vi "rename channel test.vi"() -> ()   [LabVIEW 2013, in "current tag file io module tests.lvlib"]
uses:
  current tag file io module tests.lvlib
  module/configuration/tag configuration.ctl
  <vilib>/NI/Tag Bus Module Framework/channel/TBM channel.lvclass
  <vilib>/NI/Tag Bus/tag/Data Type.ctl
  module/configuration/current tag file io module configuration.lvclass/current tag file io module configuration.ctl
  <vilib>/NI/Tag Bus/tag/tag descriptor.lvclass/tag descriptor.ctl
  module/configuration/Read tags.vi
  module/configuration/current tag file io module configuration.lvclass
  <vilib>/NI/Tag Bus/tag/tag descriptor.lvclass
panel:
  out "data output 2":T1
  out "data output":T1
  out "output 2":string
  out "output":string
  out "tag select 2":T2[](array[typedef])
  out "tag select":T2[](array[typedef])
  out "no err":errorcluster
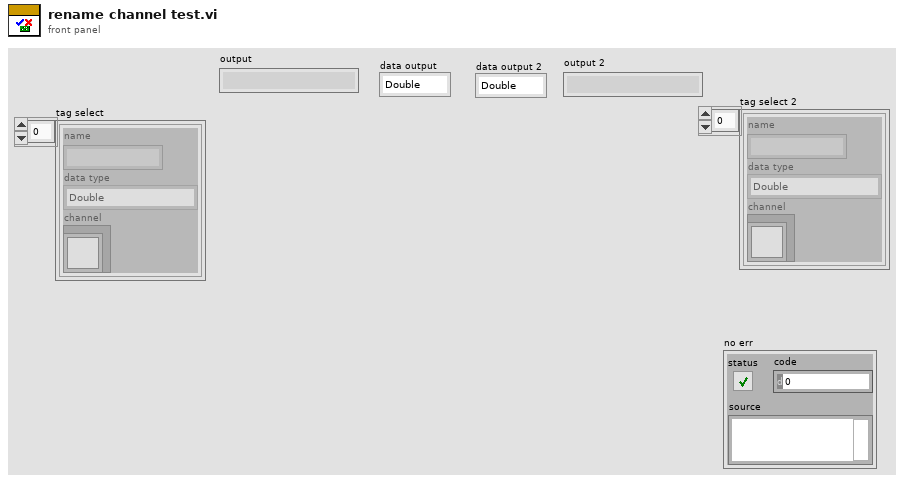
[diagram p1: front panel]
types:
  T1 = typedef "tag bus.lvlib/tag descriptor.lvclass/Data Type.ctl" = enum16{"Double", "Single", "I64", "I32", "I16", "I8", "U64", "U32", "U16", "U8", "Boolean", "String", "Array of Double", "Array of Single", "Array of I64", "Array of I32", "Array of I16", "Array of I8", "Array of U64", "Array of U32", "Array of U16", "Array of U8", "Array of Boolean", "Array of String"}
  T2 = typedef "current tag file io module configuration.lvclass/tag configuration.ctl" = cluster{"name":string, "data type":T1, "channel":refnum<class "TBM channel.lvclass">}
  T3 = typedef "current tag file io module configuration.lvclass/tag select configuration.ctl" = cluster{"name":string, "data type":T1, "channel":refnum<class "TBM channel.lvclass">}
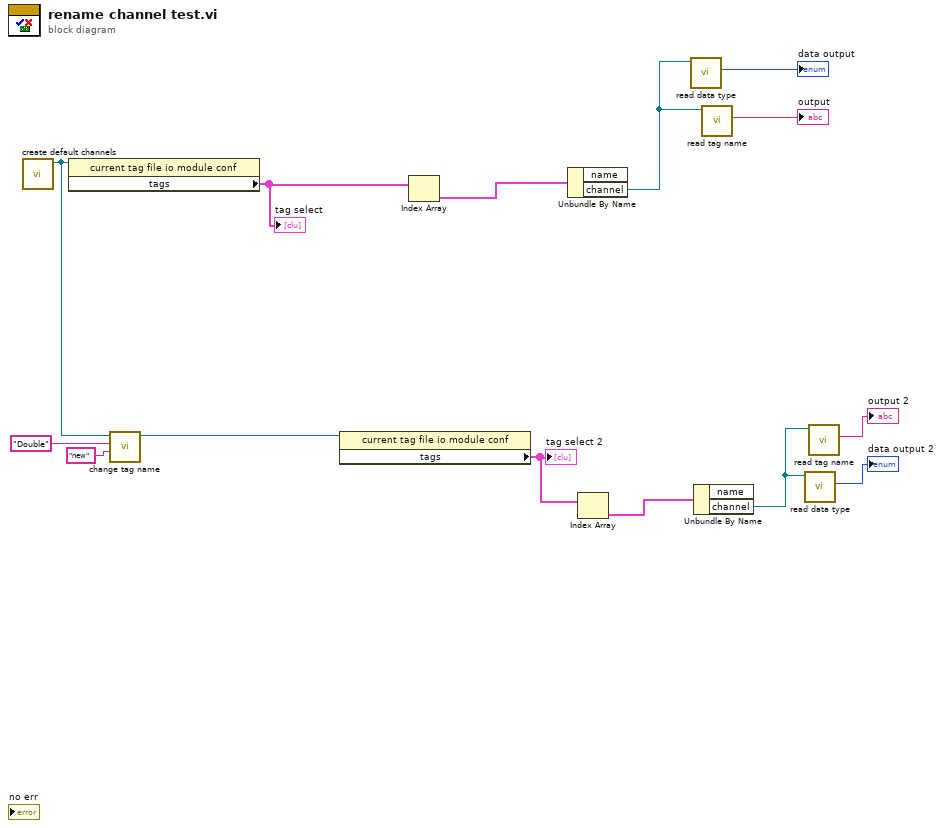
[diagram p0: block diagram]
diagram:
  n1 = call "create default channels.vi"() -> ("module"=w12:refnum<class "current tag file io module configuration.lvclass">)  [unwired: 8 in, 3 out]
  n2 = property class="current tag file io module conf"(reference=w12) -> ("tags"=w10:T3[])  [unwired: 1 in, 2 out]
  "tag select" <- w10
  n3 = call "change tag name.vi"("new name"="new", "old name"="Double", "current tag file io module configuration in"=w12) -> ("current tag file io module configuration out"=w11:refnum<class "current tag file io module configuration.lvclass">)  [unwired: 5 in, 3 out]
  n4 = property class="current tag file io module conf"(reference=w11) -> ("tags"=w5:T3[])  [unwired: 1 in, 2 out]
  "tag select 2" <- w5
  n5 = Index Array(array=w10) -> (element=w9:T3)  [unwired: 1 in]
  n6 = Unbundle By Name(w9) -> ("channel"=w3:refnum<class "TBM channel.lvclass">)  [unwired: 1 out]
  n7 = Index Array(array=w5) -> (element=w7:T3)  [unwired: 1 in]
  n8 = call <vilib>:"read data type.vi"("system tag in"=w3) -> ("data type"=→"data output":T1)  [unwired: 8 in, 2 out]
  n9 = Unbundle By Name(w7) -> ("channel"=w1:refnum<class "TBM channel.lvclass">)  [unwired: 1 out]
  n10 = call <vilib>:"read tag name.vi"("system tag in"=w3) -> ("name"=→"output":string)  [unwired: 8 in, 2 out]
  n11 = call <vilib>:"read data type.vi"("system tag in"=w1) -> ("data type"=→"data output 2":T1)  [unwired: 8 in, 2 out]
  n12 = call <vilib>:"read tag name.vi"("system tag in"=w1) -> ("name"=→"output 2":string)  [unwired: 8 in, 2 out]
